vi "MovemotorMeng.vi"(8 "error in (no error)":errorcluster, 9 "Serial number":string, 10 "Input":u32, 11 "Automation Refnum in":refnum<k7>) -> (0 "error out":errorcluster, 1 "Position":sgl, 3 "Automation Refnum out":refnum<k7>)   [LabVIEW 2014]
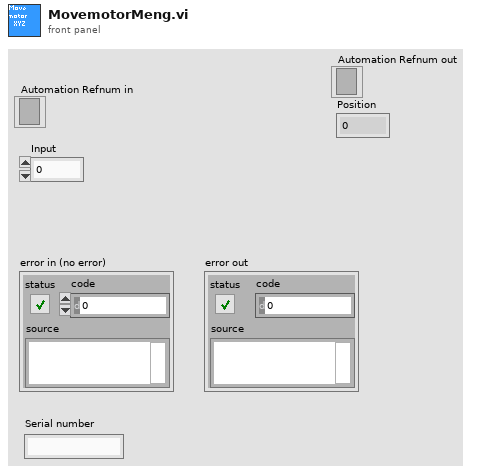
[diagram p1: front panel]
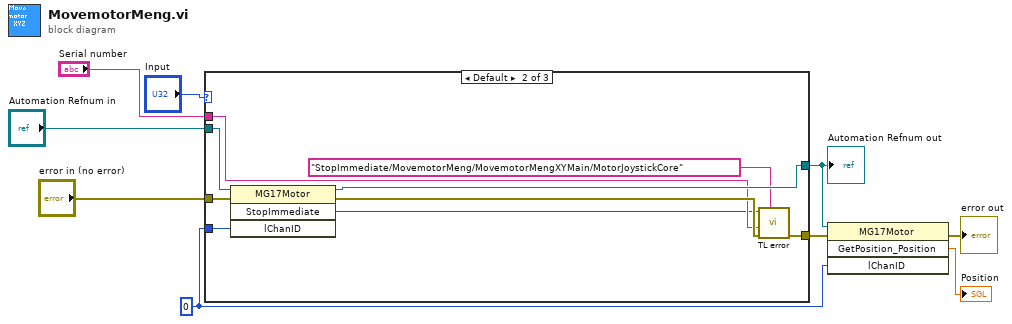
[diagram p0: block diagram]
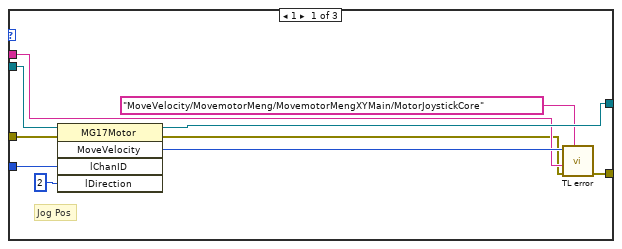
[diagram p2: hidden frame]
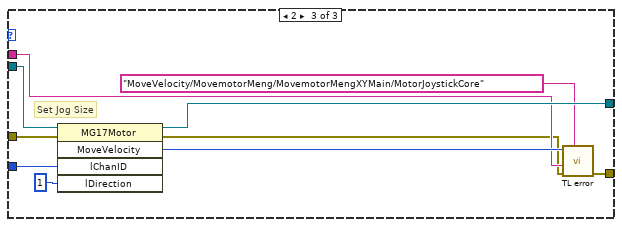
[diagram p3: hidden frame]
diagram:
  w3 = 0 ("lChanID")
  n1 = case shown="Default" "Input" {
    tunnel: "Automation Refnum in" -> [w19 w28 w38]
    tunnel: w3 -> [w18 w26 w36]
    tunnel: [w11 w23 w30] -> w1
    tunnel: "error in (no error)" -> [w17 w27 w37]
    tunnel: [w15 w25 w34] -> w6
    tunnel: "Serial number" -> [w13 w22 w32]
    frame 1 {
      # "Jog Pos"
      n2 = invoke class="MG17Motor" method="MoveVelocity"(reference=w19, error in=w17, "lChanID"=w18, "lDirection"=2) -> (reference out=w15:refnum<k7>, error out=w12:errorcluster, "MoveVelocity"=w14:i32)  [unwired: 1 in, 2 out]
      n3 = call "TL error.vi"("Input string"="MoveVelocity/MovemotorMeng/MovemotorMengXYMain/MotorJoystickCore", "error in (no error)"=w12, "Serial number of motor"=w13, "Return Code"=w14) -> ("error out"=w11:errorcluster)  [unwired: 7 in]
    }
    frame Default {
      n4 = invoke class="MG17Motor" method="StopImmediate"(reference=w28, error in=w27, "lChanID"=w26) -> (reference out=w25:refnum<k7>, error out=w24:errorcluster, "StopImmediate"=w21:i32)  [unwired: 1 in, 1 out]
      n5 = call "TL error.vi"("Input string"="StopImmediate/MovemotorMeng/MovemotorMengXYMain/MotorJoystickCore", "error in (no error)"=w24, "Serial number of motor"=w22, "Return Code"=w21) -> ("error out"=w23:errorcluster)  [unwired: 7 in]
    }
    frame 2 {
      # "Set Jog Size"
      n6 = invoke class="MG17Motor" method="MoveVelocity"(reference=w38, error in=w37, "lChanID"=w36, "lDirection"=1) -> (reference out=w34:refnum<k7>, error out=w31:errorcluster, "MoveVelocity"=w33:i32)  [unwired: 1 in, 2 out]
      n7 = call "TL error.vi"("Input string"="MoveVelocity/MovemotorMeng/MovemotorMengXYMain/MotorJoystickCore", "error in (no error)"=w31, "Serial number of motor"=w32, "Return Code"=w33) -> ("error out"=w30:errorcluster)  [unwired: 7 in]
    }
  }
  "Automation Refnum out" <- w6
  n8 = invoke class="MG17Motor" method="GetPosition_Position"(reference=w6, error in=w1, "lChanID"=w3) -> (error out=→"error out":errorcluster, "GetPosition_Position"=→"Position":sgl)  [unwired: 1 in, 2 out]
